vi "AprilTag25h9Codes.vi"() -> (0 "Codes":i64[](array[numeric])=[8987, 11941, 13418, 17849, 31142, 32619, 45912, 59205, 65113, 5485, 14347, 61611, 3460, 18230, 35954, 44816, 2364, 37812, 42243, 18063, 57655, 22421, 57154, 7197, 59868, 29613, 44383, 54576, 1994, 44846] format="%.0x", 1 "Layout":string="bbbbbbbbdddddbbdddddbbdddddbbdddddbbdddddbbbbbbbb")   [LabVIEW 2020, in "feature_detection.lvlib"]
uses:
  feature_detection.lvlib
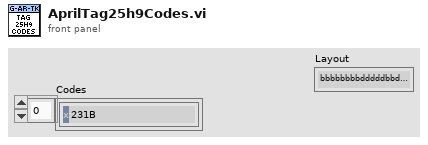
[diagram p1: front panel]
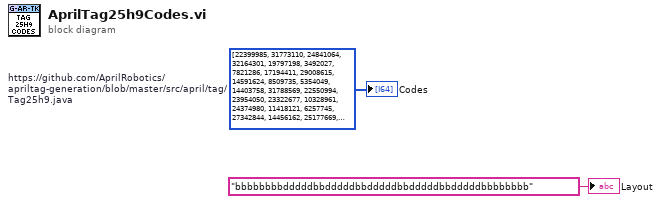
[diagram p0: block diagram]
diagram:
  w2 = i64[] [22399985, 31773110, 24841064, 32164301, 19797198, 3492027, 7821286, 17194411, 29008615, 14591624, 8509735, 5354049, 14403758, 31788569, 22550994, 23954050, 23322677, 10328961, 24374980, 11418121, 6257745, 27342844, 14456162, 25177669, 29578284, 8851364, 9520905, 23495920, 13169317, 8601275, 5861759, 20762704, 16386769, 28795824, 12161486]  # https://github.com/AprilRobotics/apriltag-generation/blob/master/src/april/tag/Tag25h9.java
  "Codes" <- w2
  "Layout" <- "bbbbbbbbdddddbbdddddbbdddddbbdddddbbdddddbbbbbbbb"
